vi "Bearing Monitor.vi"() -> ()   [LabVIEW 2023]
doc: "This example shows the application of computing the cepstrum of a signal to monitor the condition of a bearing.\n\nCepstrum analysis has many applications, such as echo cancellation and speech analysis. One of the most important applications is machine diagnosis, where you use cepstrum analysis to separate the convoluted signals and detect periodicities in the spectrum. \n\nIf you attach a sensor directly to the bearing that contains defects, you can see peaks obviously in the signal acquired by the sensor. However, you can attach sensors only to the cast shell of a machine. The cast shell that acts as a filter blurs the acquired signal. Therefore, the acquired signal is in fact a convoluted signal by the impulse response of the cast shell. You might not be able to see obvious peaks in the signal acquired from the cast shell. By computing the cepstrum, you can deconvolute the signal that the bearing generates from the impulse response of the cast shell.\n\nThis example simulates the impulse response of the cast shell with a lowpass filter and uses the TSA Real Cepstrum VI to compute the cepstrum of the signal.\n\n<b>Instructions:</b>\n1) Run this VI.\n2) Observe the cepstrum of the blurred vibration signal from the cast shell.\n3) Try different method to compute cepstrum."
uses:
  <vilib>/addons/Time Series Analysis/Utilities.llb/TSA Data.ctl
  <vilib>/Analysis/3filter.llb/Butterworth Filter (DBL).vi
  <vilib>/addons/Time Series Analysis/Correlation and Spectral Analysis.llb/TSA Real Cepstrum (Waveform).vi
  <vilib>/addons/_Advanced Signal Processing/NI_AdvSigProcTSA.lvlib
  <vilib>/Analysis/NI_AALBase.lvlib
panel:
  in  "stop":bool
  in  "AR order":i32=40
  in  "Method":u16(ring)=1 items=["FFT", "AR Model"]
  in  "Cepstrum bins":i32=256
  out "Cepstrum of Blurred Vibration":cluster{"t0":dbl, "dt":dbl, "C(t)":dbl[]}(graph)
  out "Vibration Blurred by Cast Shell":waveform(dbl)(graph)
  out "Original Vibration":waveform(dbl)(graph)
  # "Overview: Shows the application of computing the cepstrum of a signal to monitor the condition of a bearing.\nRequirements: LabVIEW Full Development System, Advanced Signal Processing Toolkit\nInstructions: \n1. Run this VI.\n2. Observe the cepstrum of the blurred vibration signal from the cast shell.\n3. Change the settings in the Settings of Cepstrum Computation to compute cepstrum.\n4. Click Stop to stop the VI."
  # "Settings of Cepstrum Computation"
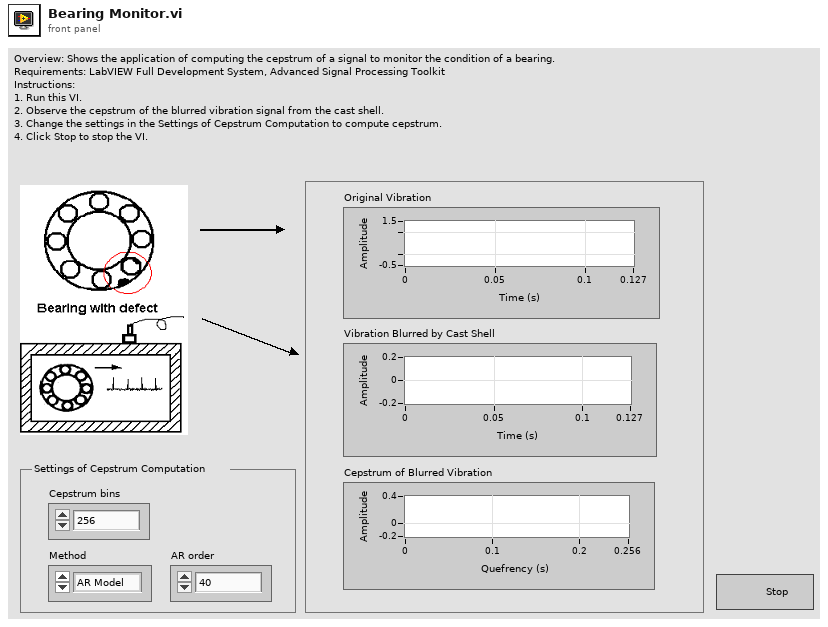
[diagram p1: front panel]
types:
  T1 = enum32{"Lowpass", "Highpass", "Bandpass", "Bandstop"}
  T2 = typedef "NI_AdvSigProcTSA.lvlib/TSA Data.ctl" = u16
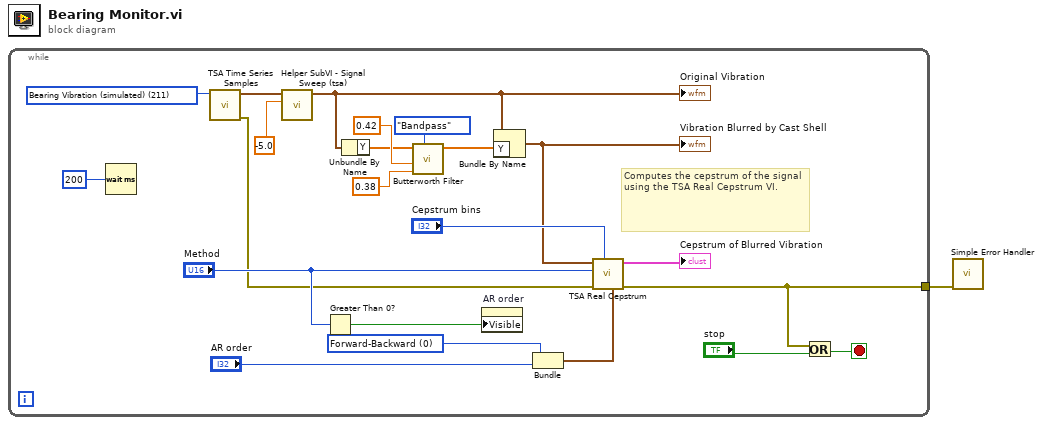
[diagram p0: block diagram]
diagram:
  n1 = while {
    tunnel: [w3] -> w1
    stop <- w12 stop-if-true
    w4 = T2 211 items=["Kobe Earthquake"=201, "EEG"=210, "Bearing Vibration (simulated)"=211, "Period Product Sales"=214, "Beam Vibration (nonlinear)"=217, "Beam Vibration (linear)"=218, "Signal With Echo"=219, "Engine Knocking"=220, "Power Line"=221, "-"=200, "Beam Deflections (multivariate)"=207, "Structure Vibration (multivariate)"=208, "Human MEG (multivariate)"=222] ("data")
    w14 = u16 0 items=["Forward-Backward", "Least-Squares", "Yule-Walker", "Burg-Lattice", "Geometric-Lattice"] ("method")
    # "Computes the cepstrum of the signal using the TSA Real Cepstrum VI."
    n2 = Wait (ms)(milliseconds to wait=u32 200 ("millisecond multiple")) -> ()  [unwired: 1 out]
    n3 = call <vilib>:"TSA Time Series Samples.vi"("data"=w4) -> ("error out"=w2:errorcluster, "univariate time series"=w9:waveform(dbl))  [unwired: 1 in, 8 out]
    n4 = call "Helper SubVI - Signal Sweep (tsa).vi"("shift (%)"=-5.0, "Signal in"=w9) -> ("Signal out"=w6:waveform(dbl))  [unwired: 9 in]
    "Original Vibration" <- w6
    n5 = Greater Than 0?(x="Method") -> (x > 0?=w17:bool)
    n6 = Unbundle By Name(w6) -> ("Y"=w8:dbl[])
    n7 = call-poly <vilib>:"Butterworth Filter.vi"("filter type"=T1."Bandpass", "low cutoff freq: fl"=0.38, "high cutoff freq: fh"=0.42, "X"=w8) -> ("Filtered X"=w7:dbl[])  [unwired: 3 in, 2 out]
    n8 = property on="AR order" class="DigNum (strict)"("Visible"=w17) -> ()  [unwired: 2 in, 2 out]
    n9 = Bundle By Name(cluster=w6, "Y"=w7) -> (w5:waveform(dbl))
    "Vibration Blurred by Cast Shell" <- w5
    n10 = Bundle("method"=w14, "AR order"="AR order") -> (w15:cluster{"method":u16, "AR order":i32})  [unwired: 1 out]
    n11 = call-poly <vilib>:"TSA Real Cepstrum.vi"("AR setting"=w15, "cepstrum bins"="Cepstrum bins", "error in (no error)"=w2, "method"="Method", "Xt"=w5) -> ("error out"=w3:errorcluster, "cepstrum"=→"Cepstrum of Blurred Vibration":cluster{"t0":dbl, "dt":dbl, "C(t)":dbl[]})  [unwired: 1 in, 4 out]
    n12 = Or(x=w3, y="stop") -> (x .or. y?=w12:bool)
  }
  n13 = call <vilib>:"Simple Error Handler.vi"("error in (no error)"=w1) -> ()  [unwired: 1 in, 8 out]
